vi "_SetHubPort.vi"(8 "error in":errorcluster, 10 "HubPort":i32, 11 "Device In":u64) -> (0 "error out":errorcluster, 3 "Device Out":u64)   [LabVIEW 2012, in "Phidget Common.lvlib"]
uses:
  <instrlib>/Phidgets/Phidget Common/Phidget Common.lvlib
  phidget22.dll
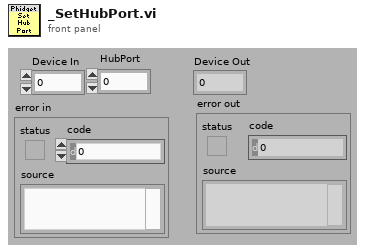
[diagram p1: front panel]
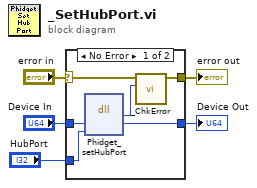
[diagram p0: block diagram]
diagram:
  n1 = case shown="No Error" "error in" {
    selector: "error in" -> [w9 w13]
    tunnel: [w7 w13] -> w4
    tunnel: "Device In" -> [w11 w12]
    tunnel: [w10 w12] -> w2
    tunnel: "HubPort" -> [w6 _]
    frame No Error {
      n2 = dll-call lib="phidget22.dll" fn="Phidget_setHubPort"("phid"=w11, "HubPort"=w6) -> ("return type"=w8:i32, "phid"=w10:u64)  [unwired: 4 in, 2 out]
      n3 = call <instrlib>:"_ChkError.vi"("Return Code"=w8, "error in (no error)"=w9) -> ("error out"=w7:errorcluster)  [unwired: 9 in]
    }
    frame Error {
    }
  }
  "error out" <- w4
  "Device Out" <- w2
